vi "set current activity.vi"(8 "error in (no error)":errorcluster, 10 "Current activity":T1=enum."Idle", 11 "Autofocus in":refnum<class "Autofocus.lvclass">) -> (0 "error out":errorcluster, 3 "Autofocus out":refnum<class "Autofocus.lvclass">)   [LabVIEW 2012, in "Autofocus.lvclass"]
uses:
  Autofocus.lvclass
  current activity.ctl
  Autofocus.lvclass/Autofocus.ctl
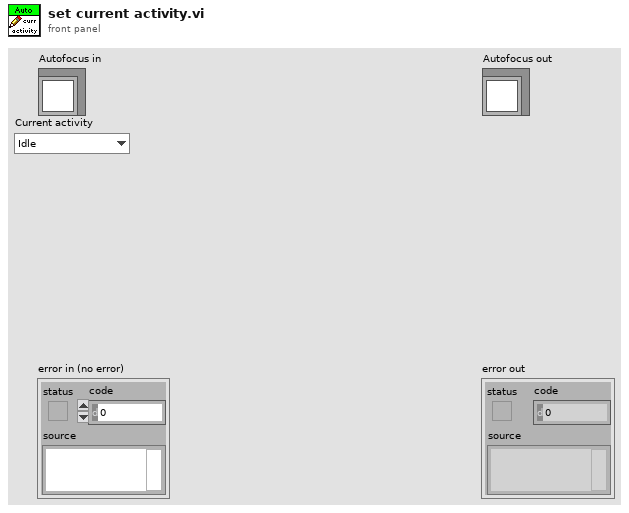
[diagram p1: front panel]
types:
  T1 = typedef "Autofocus.lvclass/current activity.ctl" = enum16{"Image acquisition", "Stack", "Checkpoint", "Idle"}
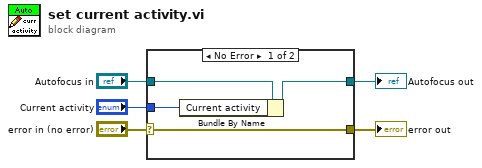
[diagram p0: block diagram]
diagram:
  n1 = case shown="No Error" "error in (no error)" {
    selector: "error in (no error)" -> [w9 w11]
    tunnel: [w9 w11] -> w4
    tunnel: [w7 w10] -> w2
    tunnel: "Autofocus in" -> [w8 w10]
    tunnel: "Current activity" -> [w6 _]
    frame No Error {
      n2 = Bundle By Name(cluster=w8, "Current activity"=w6) -> (w7:refnum<class "Autofocus.lvclass">)
    }
    frame Error {
    }
  }
  "error out" <- w4
  "Autofocus out" <- w2
